vi "PH_gentec_M-Link.Data Flow.vi"(0 "i ref in":refnum<vi>, 2 "VISA resource in":refnum<visa-resource-name>, 3 "Data Flow State to set":bool, 5 "error in":errorcluster) -> (14 "i ref out":refnum<vi>, 15 "Error":bool, 16 "Failure":bool, 17 "Data Read":string[](array[string]), 18 "Read Timeout":bool, 19 "error out":errorcluster)   [LabVIEW 2014, in "PH_gentec_M-Link.lvlib"]
doc: "This VI sets the Data Flow to the State connected to \"Data Flow to set\"."
uses:
  PH_gentec_M-Link.lvlib
  instr.lib/Gentec-M-Link/gentec-M-Link - Driver.lvlib
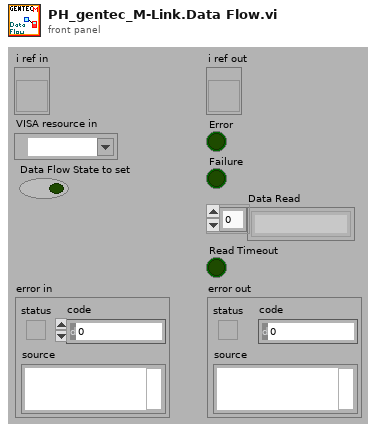
[diagram p1: front panel]
types:
  T1 = typedef "PH_gentec_M-Link.lvlib/PH_gentec_M-Link.i attribute.ctl" = cluster{"GUI References":cluster{"Wanted Head Settings":refnum<vi>, "Current Head Settings":refnum<vi>, "Set Auto Range":refnum<vi>, "Trigger Polarity":refnum<vi>, "Trigger Source":refnum<vi>, "Waveform Averages":refnum<vi>, "Continuous":refnum<vi>, "get one Value":refnum<vi>}, "Wanted Head Settings":T2, "Current Head Settings":T2}
  T2 = typedef "PH_gentec_M-Link.lvlib/PH_gentec_M-Link.Head Settings.ctl" = cluster{"Measurement Mode":T3, "Enable Anticipation":bool, "Set Auto Range":bool, "Block Signal":bool, "Set Head Attenuator":bool, "Enable SSE":bool, "Trigger Polarity":T4, "Trigger Source":T5, "Waveform Averages":T6, "Set Zero":i32, "Current Measurement":i32, "Start Data Flow":bool}
  T3 = typedef "gentec-M-Link - Driver.lvlib/gentec-M-Link.Measurement Mode.ctl" = u16
  T4 = typedef "gentec-M-Link - Driver.lvlib/gentec-M-Link.Trigger Polarity.ctl" = u16
  T5 = typedef "gentec-M-Link - Driver.lvlib/gentec-M-Link.Trigger Source.ctl" = u16
  T6 = typedef "gentec-M-Link - Driver.lvlib/gentec-M-Link.Waveform Averages.ctl" = u16
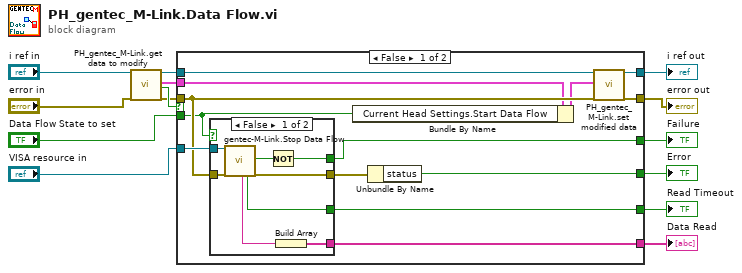
[diagram p0: block diagram]
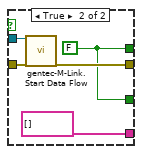
[diagram p2: hidden frame]
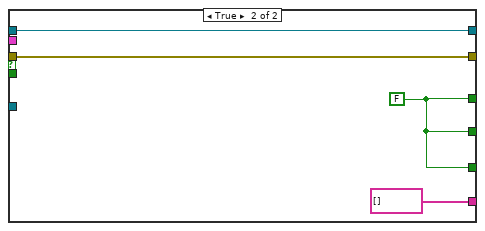
[diagram p3: hidden frame]
diagram:
  n1 = call "PH_gentec_M-Link.get data to modify.vi"("i ref in"="i ref in", "error in (no error)"="error in") -> ("i ref out"=w5:refnum<vi>, "i attribute"=w6:T1, "timed out"=w7:bool, "error out"=w4:errorcluster)  [unwired: 14 in]
  n2 = case shown="False" w7 {
    tunnel: "VISA resource in" -> [w26 _]
    tunnel: [w23 w44] -> w2
    tunnel: [w22 w43] -> w1
    tunnel: w4 -> [w25 w43]
    tunnel: w5 -> [w27 w44]
    tunnel: w6 -> [w24 _]
    tunnel: "Data Flow State to set" -> [w18 _]
    tunnel: [w20 w42] -> w11
    tunnel: [w16 w42] -> w12
    tunnel: [w17 w42] -> w13
    tunnel: [w15 string[] []] -> w14
    frame False {
      n3 = case shown="False" w18 {
        tunnel: w26 -> [w35 w40]
        tunnel: w25 -> [w34 w39]
        tunnel: [w33 w38] -> w19
        tunnel: [w30 w37] -> w16
        tunnel: [w31 w37] -> w17
        tunnel: [w28 string[] []] -> w15
        frame False {
          n4 = call "gentec-M-Link.Stop Data Flow.vi"("VISA resource In"=w35, "error in (no error)"=w34) -> ("Data Read"=w29:string, "Read Timeout"=w31:bool, "Success"=w32:bool, "error out"=w33:errorcluster)  [unwired: 13 in, 1 out]
          n5 = Not(x=w32) -> (.not. x?=w30:bool)
          n6 = Build Array(w29) -> (w28:string[])
        }
        frame True {
          w37 = FALSE
          n7 = call "gentec-M-Link.Start Data Flow.vi"("VISA resource In"=w40, "error in (no error)"=w39) -> ("error out"=w38:errorcluster)  [unwired: 16 in, 1 out]
        }
      }
      n8 = Bundle By Name(cluster=w24, "Current Head Settings.Start Data Flow"=w18) -> (w21:T1)
      n9 = Unbundle By Name(w19) -> ("status"=w20:bool)
      n10 = call "PH_gentec_M-Link.set modified data.vi"("i ref in"=w27, "i attribute"=w21, "error in (no error)"=w25) -> ("i ref out"=w23:refnum<vi>, "error out"=w22:errorcluster)  [unwired: 15 in]
    }
    frame True {
      w42 = FALSE
    }
  }
  "Data Read" <- w14
  "Read Timeout" <- w13
  "Failure" <- w12
  "Error" <- w11
  "i ref out" <- w2
  "error out" <- w1
